vi "Green_XOR_Filter.vi"(0 "Image Src 1":T1, 1 "Processed 1 Dst":T1, 2 "Image Src 2":T1, 3 "Processed 2 Dst":T1, 5 "XOR Dst":T1, 7 "Green Range":cluster{"Lower value":i32, "Upper value":i32}={"Lower value"=0, "Upper value"=255}) -> (15 "XOR Image":T1, 17 "Processed Image 1":T1, 18 "Processed Image 2":T1)   [LabVIEW 2011]
uses:
  <vilib>/vision/Image Controls.llb/IMAQ Image.ctl
  <vilib>/vision/NI_Vision_Development_Module.lvlib
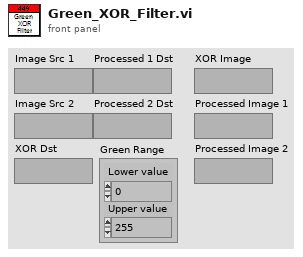
[diagram p1: front panel]
types:
  T1 = typedef "IMAQ Image.ctl" = refnum<image>
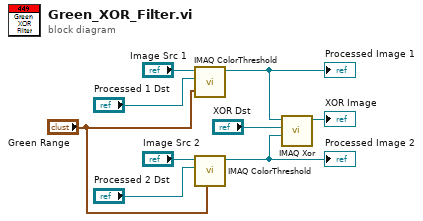
[diagram p0: block diagram]
diagram:
  n1 = call "IMAQ ColorThreshold"("Green or Sat Range"="Green Range", "Image Dst"="Processed 1 Dst", "Image Src"="Image Src 1") -> ("Image Dst Out"=w2:T1)  [unwired: 7 in, 1 out]
  "Processed Image 1" <- w2
  n2 = call "IMAQ ColorThreshold"("Green or Sat Range"="Green Range", "Image Dst"="Processed 2 Dst", "Image Src"="Image Src 2") -> ("Image Dst Out"=w1:T1)  [unwired: 7 in, 1 out]
  "Processed Image 2" <- w1
  n3 = call "IMAQ Xor"("Image Src B"=w1, "Image Dst"="XOR Dst", "Image Src A"=w2) -> ("Image Dst Out"=→"XOR Image":T1)  [unwired: 7 in, 1 out]
